vi "QCP_Get_I32_Array.vi"(0 "Data Value Reference in":T1, 1 "String":string, 3 "error in (no error)":errorcluster) -> (7 "Data Value Reference Out":T1, 8 "Array":i32[](array[numeric]), 10 "Error Out":errorcluster)   [LabVIEW 2015]
uses:
  <userlib>/836-Library/System/QCP Support Code/QCP Data Block.ctl
  <userlib>/836-Library/System/QCP Support Code/QCP_Get_I32.vi
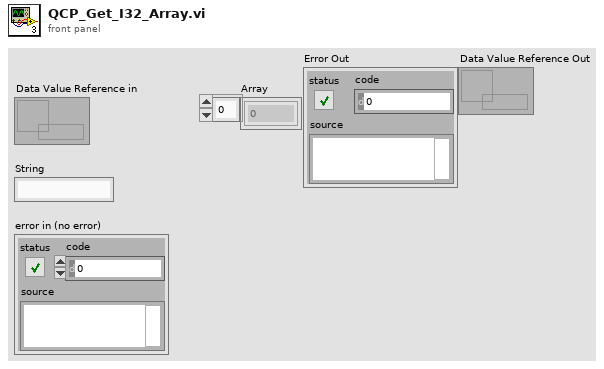
[diagram p1: front panel]
types:
  T1 = typedef "QCP Data Block.ctl" = refnum<data-value>
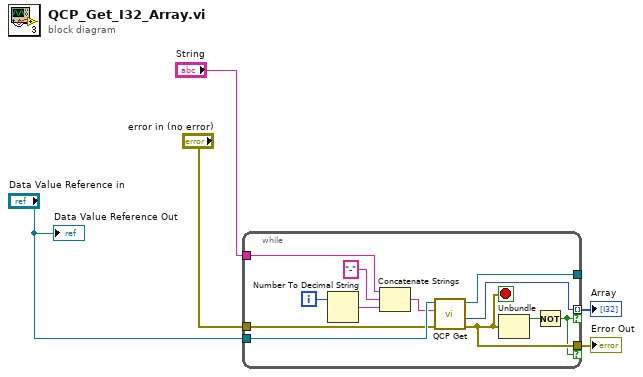
[diagram p0: block diagram]
diagram:
  n1 = while {
    tunnel: "String" -> [w17]
    tunnel: "Data Value Reference in" -> [w16]
    tunnel: [w12] -> w5 mode=indexing if=w6
    tunnel: [w11] -> _
    tunnel: "error in (no error)" -> [w10]
    tunnel: [w7] -> w1 if=w6
    i -> [w9]
    stop <- w7 stop-if-true
    n2 = Number To Decimal String(number=w9) -> (decimal integer string=w14:string)  [unwired: 1 in]
    n3 = Concatenate Strings(w17, "-" ("string"), w14) -> (w13:string)
    n4 = call-poly <userlib>:"QCP Get.vi"("QCP Data Block In"=w16, "QCP Name"=w13, "Error In"=w10) -> ("QCP Data Block Out"=w11:T1, "Value Out"=w12:i32, "Error Out"=w7:errorcluster)  [unwired: 5 in]
    n5 = Unbundle(w7) -> ("status"=w8:bool)  [unwired: 2 out]
    n6 = Not(x=w8) -> (.not. x?=w6:bool)
  }
  "Array" <- w5
  "Error Out" <- w1
  "Data Value Reference Out" <- "Data Value Reference in"
